vi "OE1022D_Configure Input Filter.vi"(0 "VISA resource name":refnum<visa-resource-name>, 1 "Input Source":u16(ring) format="%x" items=["Single-Ended Voltage", "Differential Voltage", "1 MOhm Current Gain", "100 MOhm Current Gain"], 2 "Input Shield Grounding":u8(ring) items=["Float", "Ground"], 5 "OE1022D A/B":u8(ring) items=["Channel A", "Channel B"], 11 "error in (no error)":errorcluster, 12 "Input Coupling":u8(ring) items=["AC", "DC"], 13 "Input Notch Filter":u8(ring) items=["None", "Line Notch", "Both Notch Filters", "2x Line Notch"]) -> (4 "VISA resource name out":refnum<visa-resource-name>, 15 "error out":errorcluster)   [LabVIEW 2024]
doc: "Configures the reference source and the internal oscillator."
panel:
  # "Signal Generator"
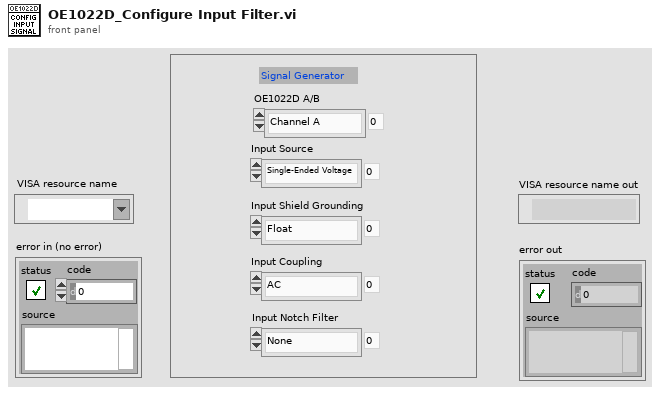
[diagram p1: front panel]
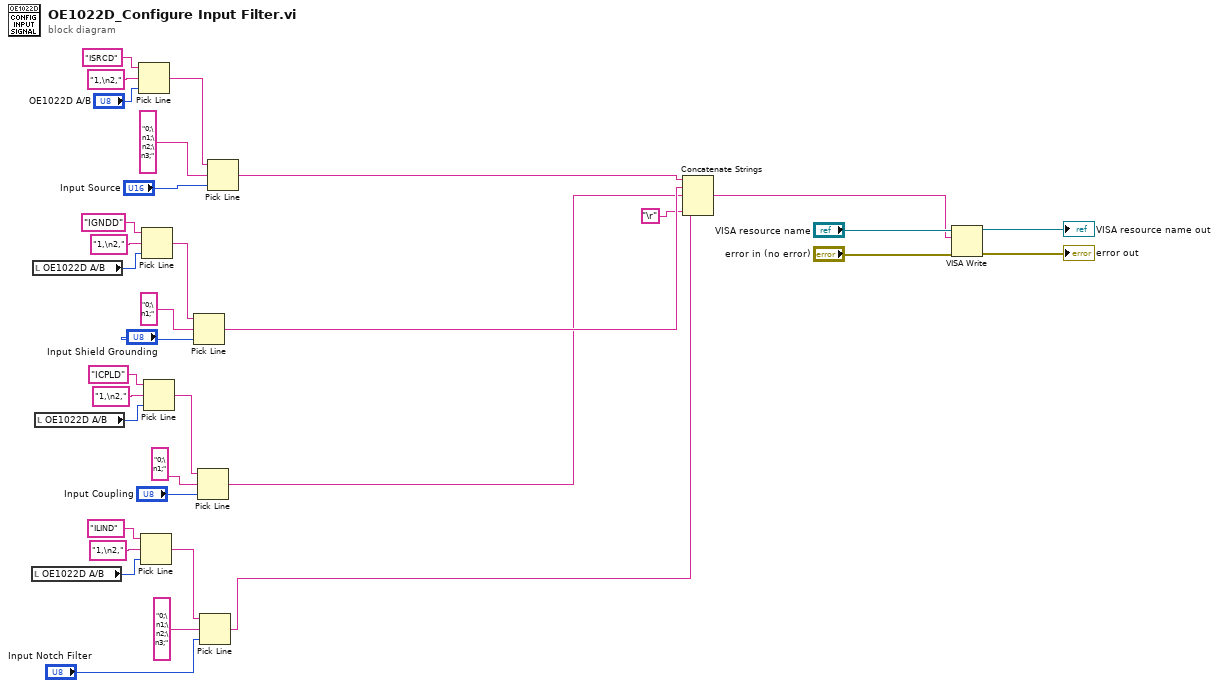
[diagram p0: block diagram]
diagram:
  n1 = local read "OE1022D A/B"() -> (w6:u8)
  n2 = local read "OE1022D A/B"() -> (w15:u8)
  n3 = local read "OE1022D A/B"() -> (w12:u8)
  n4 = Pick Line(string ("")="ISRCD", multi-line string="1,\n2,", line index="OE1022D A/B") -> (output string=w19:string)
  n5 = Pick Line(string ("")="ILIND", multi-line string="1,\n2,", line index=w6) -> (output string=w5:string)
  n6 = Pick Line(string ("")="IGNDD", multi-line string="1,\n2,", line index=w15) -> (output string=w14:string)
  n7 = Pick Line(string ("")="ICPLD", multi-line string="1,\n2,", line index=w12) -> (output string=w9:string)
  n8 = Pick Line(string ("")=w14, multi-line string="0;\n1;", line index="Input Shield Grounding") -> (output string=w13:string)
  n9 = Pick Line(string ("")=w9, multi-line string="0;\n1;", line index="Input Coupling") -> (output string=w4:string)
  n10 = Pick Line(string ("")=w5, multi-line string="0;\n1;\n2;\n3;", line index="Input Notch Filter") -> (output string=w3:string)
  n11 = Pick Line(string ("")=w19, multi-line string="0;\n1;\n2;\n3;", line index="Input Source") -> (output string=w18:string)
  n12 = Concatenate Strings(w18, w13, w4, w3, "\r") -> (w1:string)
  n13 = VISA Write(VISA resource name="VISA resource name", write buffer=w1, error in (no error)="error in (no error)") -> (VISA resource name out=→"VISA resource name out":refnum<visa-resource-name>, error out=→"error out":errorcluster)  [unwired: 1 out]
